vi "Delete Junk Data.vi"(10 "DAQ Array":dbl[](array[numeric]), 11 "Newfi Input Array":dbl[](array[numeric])) -> (1 "DAQ Array Output":dbl[](array[numeric]), 2 "Deleted Rows":i32[](array[numeric]), 3 "Data":dbl[](array[numeric]))   [LabVIEW 2016]
uses:
  <vilib>/gmath/statdist.llb/st_Percentiles (scalar).vi
  <vilib>/gmath/NI_Gmath.lvlib
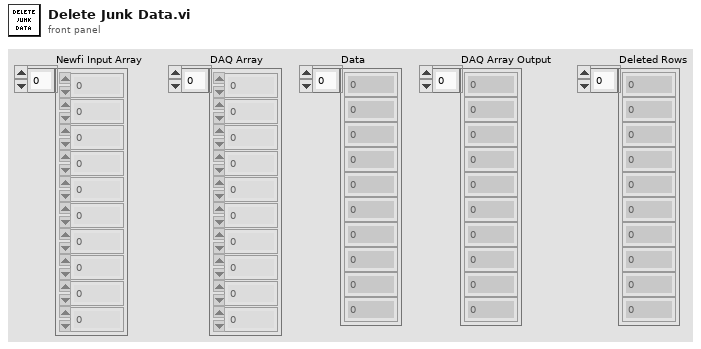
[diagram p1: front panel]
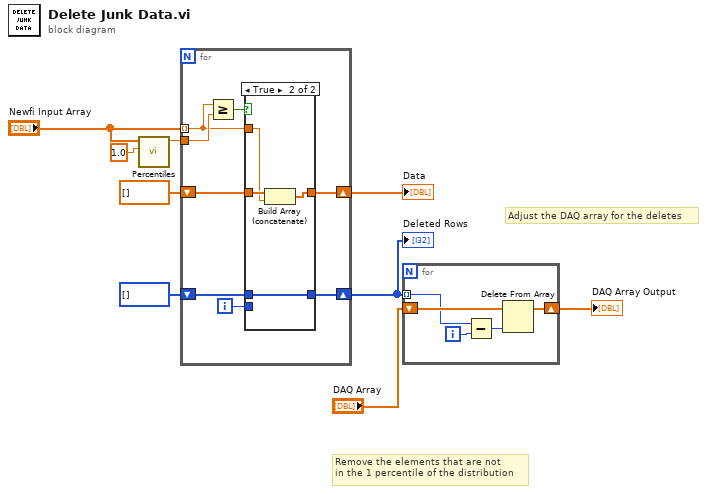
[diagram p0: block diagram]
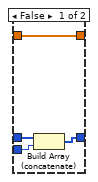
[diagram p2: hidden frame]
diagram:
  # "Adjust the DAQ array for the deletes"
  # "Remove the elements that are not\nin the 1 percentile of the distribution"
  n1 = call-poly <vilib>:"Percentiles.vi"("p"=1.0, "x array"="Newfi Input Array") -> ("percentile"=w7:dbl)  [unwired: 8 in, 1 out]
  n2 = for {
    tunnel: "Newfi Input Array" -> [w14] mode=indexing
    tunnel: w7 -> [w17]
    shift-right: [w13] -> w9
    shift-left: dbl[] [] -> [w15]
    shift-right: [w10] -> w3
    shift-left: i32[] [] -> [w12]
    i -> [w11]
    n3 = Greater Or Equal?(x=w14, y=w17) -> (x >= y?=w16:bool)
    n4 = case shown="True" w16 {
      tunnel: w15 -> [w21 w25]
      tunnel: w14 -> [_ w24]
      tunnel: [w21 w23] -> w13
      tunnel: w12 -> [w20 w22]
      tunnel: w11 -> [w19 _]
      tunnel: [w18 w22] -> w10
      frame False {
        n5 = Build Array (concatenate)(w20, w19) -> (w18:i32[])
      }
      frame True {
        n6 = Build Array (concatenate)(w25, w24) -> (w23:dbl[])
      }
    }
  }
  "Deleted Rows" <- w3
  "Data" <- w9
  n7 = for {
    tunnel: w3 -> [w29] mode=indexing
    shift-right: [w26] -> w1
    shift-left: "DAQ Array" -> [w30]
    i -> [w28]
    n8 = Subtract(x=w29, y=w28) -> (x-y=w27:i32)
    n9 = Delete From Array(array=w30, index=w27) -> (array with subset deleted=w26:dbl[])  [unwired: 1 in, 1 out]
  }
  "DAQ Array Output" <- w1
